vi "Create SecureDenyPubCircles Profile.vi"(7 "DomainParticipant Base Profile Name":string="LabVIEWLibrary::NoTypeCodeProfile", 8 "error in (no error)":errorcluster, 11 "New Custom Secure Profile Name":string="SecureDenyPubCircles") -> (0 "error out":errorcluster, 3 "Custom Secure Profile Name Output":string)   [LabVIEW 2012]
doc: "Add the options of PEER2 to the provided base Secure Profile. This PEER2 configuration denies to publish Circles."
uses:
  RTI/GIT_HEAD/connextdds/lvdds.1.0/srcLV/lvdds.1.0_package/Types/RTI DDS Security Settings.ctl
  RTI/GIT_HEAD/connextdds/lvdds.1.0/srcLV/lvdds.1.0_package/Types/RTI DDS Basic Security Settings.ctl
  RTI/GIT_HEAD/connextdds/lvdds.1.0/srcLV/lvdds.1.0_package/Types/RTI DDS Advanced Security Settings.ctl
  RTI/GIT_HEAD/connextdds/lvdds.1.0/srcLV/lvdds.1.0_package/Library/LVDDS_library.lvlib
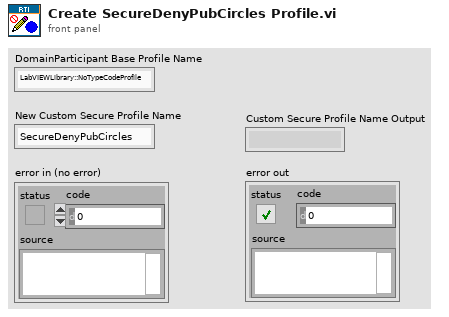
[diagram p1: front panel]
types:
  T1 = typedef "LVDDS_library.lvlib/RTI DDS Basic Security Settings.ctl" = cluster{"Identity Certificate Authority (CA)":path, "Identity Certificate (Signed by Identity CA)":path, "Private Key":path, "Permissions Certificate Authority (CA)":path, "Governance Document (Signed by Permissions CA)":path, "Permissions Document (Signed by Permissions CA)":path}
  T2 = typedef "LVDDS_library.lvlib/RTI DDS Security Settings.ctl" = cluster{"Basic Security Settings":T1, "Advanced Security Settings":T3}
  T3 = typedef "LVDDS_library.lvlib/RTI DDS Advanced Security Settings.ctl" = cluster{"Shared Secret Algorithm":string, "Encryption Algorithm":string, "Certificate Revocation List":path}
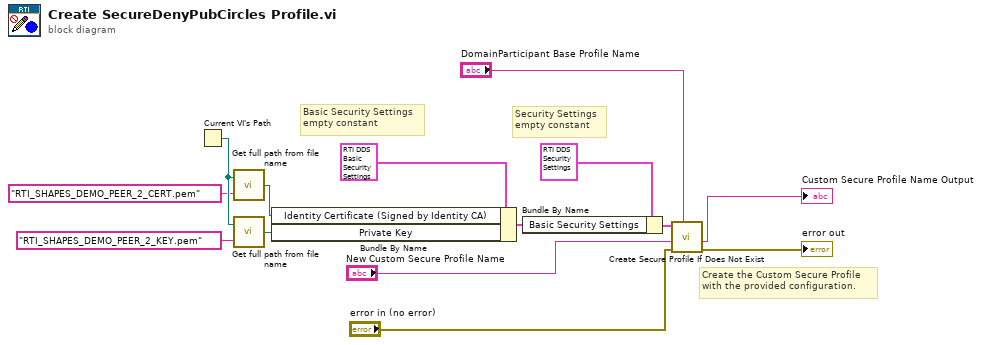
[diagram p0: block diagram]
diagram:
  # "Security Settings \nempty constant"
  # "Basic Security Settings \nempty constant"
  # "Create the Custom Secure Profile\nwith the provided configuration."
  n1 = Current VI's Path() -> (path=w14:path)
  n2 = call "Get full path from file name.vi"("File Name"="RTI_SHAPES_DEMO_PEER_2_CERT.pem", "Current Path"=w14) -> ("Full Path"=w11:path)
  n3 = call "Get full path from file name.vi"("File Name"="RTI_SHAPES_DEMO_PEER_2_KEY.pem", "Current Path"=w14) -> ("Full Path"=w8:path)
  n4 = Bundle By Name(cluster=T1 {"Identity Certificate Authority (CA)"=path "", "Identity Certificate (Signed by Identity CA)"=path "", "Private Key"=path "", "Permissions Certificate Authority (CA)"=path "", "Governance Document (Signed by Permissions CA)"=path "", "Permissions Document (Signed by Permissions CA)"=path ""} ("Basic Security Settings"), "Identity Certificate (Signed by Identity CA)"=w11, "Private Key"=w8) -> (w12:T1)
  n5 = Bundle By Name(cluster=T2 {"Basic Security Settings"={"Identity Certificate Authority (CA)"=path "", "Identity Certificate (Signed by Identity CA)"=path "", "Private Key"=path "", "Permissions Certificate Authority (CA)"=path "", "Governance Document (Signed by Permissions CA)"=path "", "Permissions Document (Signed by Permissions CA)"=path ""}, "Advanced Security Settings"={"Shared Secret Algorithm"="ecdsa-ecdh", "Encryption Algorithm"="aes-128-gcm", "Certificate Revocation List"=path ""}} ("Security Settings"), "Basic Security Settings"=w12) -> (w3:T2)
  n6 = call "Create Secure Profile If Does Not Exist.vi"("Base Profile"="DomainParticipant Base Profile Name", "error in (no error)"="error in (no error)", "New Profile Name"="New Custom Secure Profile Name", "Security Settings"=w3) -> ("error out"=→"error out":errorcluster, "New Profile Name Output"=→"Custom Secure Profile Name Output":string)  [unwired: 6 in]
